vi "Destroy.vi"(8 "error in (no error)":errorcluster, 11 "Subsequence in":refnum<class "Subsequence.lvclass">) -> (0 "error out":errorcluster)   [LabVIEW 2020, in "Test Executive.lvlib" / "Subsequence.lvclass"]
uses:
  <vilib>/gpm_packages/@cs/test-executive/Source/Test Executive/Subsequence/Subsequence.lvclass
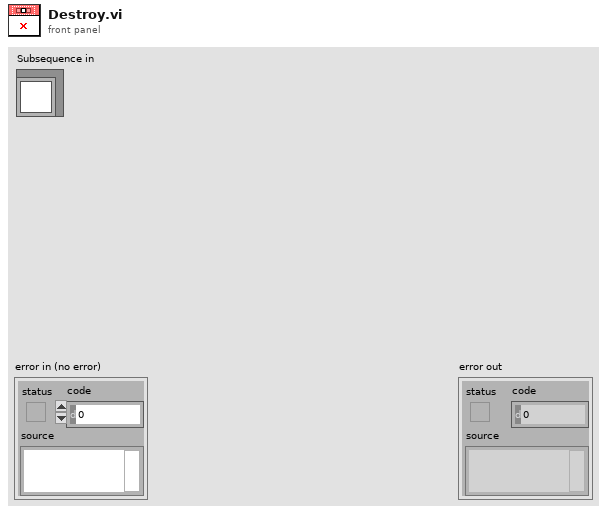
[diagram p1: front panel]
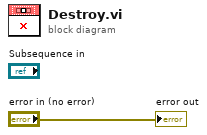
[diagram p0: block diagram]
diagram:
  "error out" <- "error in (no error)"
